vi "PS get status.vi"(8 "error in (no error)":errorcluster, 9 "Reset":bool, 11 "VISA Resource Name":refnum<visa-resource-name>) -> (0 "error out":errorcluster, 1 "Setpoint":dbl format="%.2f", 2 "Current":dbl(slide)=6.428571428571429 scale=-20.0..20.0 scale format="%.1f", 3 "dup VISA Resource Name":refnum<visa-resource-name>, 4 "Errors Out":string[](array[string]), 5 "Commands Out":string[](array[string]), 6 "% errors":dbl format="%.2f", 7 "Status":T1)   [LabVIEW 2020]
panel:
  out "Serial time":i32
  in  "samples lp filter":dbl
  out "execution time":dbl format="%.2f"
  out "# Errors":i32
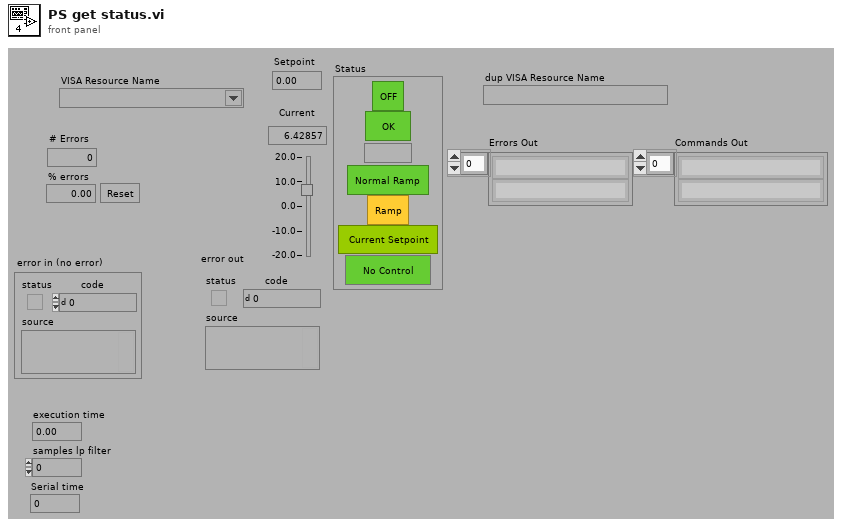
[diagram p1: front panel]
types:
  T1 = cluster{bool, bool, "Ramp Status":u16, bool, bool, bool, bool}
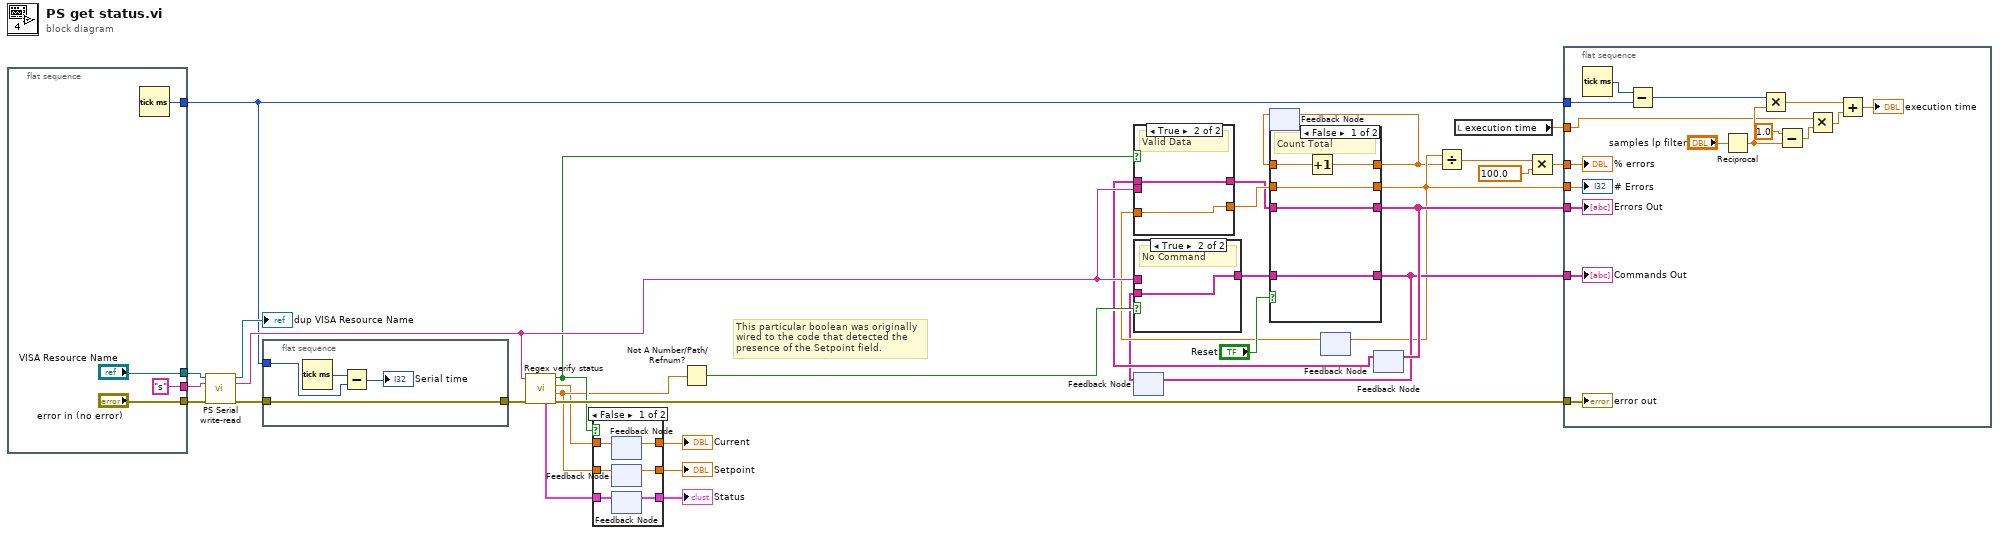
[diagram p0: block diagram]
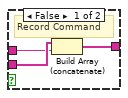
[diagram p2: hidden frame]
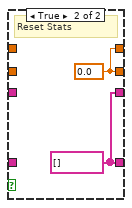
[diagram p3: hidden frame]
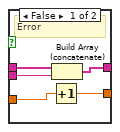
[diagram p4: hidden frame]
diagram:
  # "This particular boolean was originally\nwired to the code that detected the\npresence of the Setpoint field."
  n1 = flat-sequence {
    tunnel: ["s" ("String To Send")] -> w29
    tunnel: ["error in (no error)"] -> w28
    tunnel: ["VISA Resource Name"] -> w27
    tunnel: [w34] -> w20
    frame #0 {
      n2 = Tick Count (ms)() -> (millisecond timer value=w34:u32)
    }
  }
  n3 = call "PS Serial write-read.vi"("VISA Resource Name"=w27, "String To Send"=w29, "error in (no error)"=w28) -> ("dup VISA Resource Name"=→"dup VISA Resource Name":refnum<visa-resource-name>, "Serial Read"=w25:string, "error out"=w19:errorcluster)  [unwired: 8 in, 2 out]
  n4 = flat-sequence {
    tunnel: w20 -> [w39]
    tunnel: w19 -> [w38]
    tunnel: [w38] -> w18
    frame #0 {
      n5 = Tick Count (ms)() -> (millisecond timer value=w40:u32)
      n6 = Subtract(x=w40, y=w39) -> (x-y=→"Serial time":u32)
    }
  }
  n7 = call "Regex verify status.vi"("Error In"=w18, "Input String"=w25) -> ("Error Out"=w24:errorcluster, "Setpoint/Rate"=w4:dbl, "Current"=w2:dbl, "Valid Data"=w23:bool, "Status"=w6:T1)  [unwired: 5 in]
  n8 = case shown="False" w23 {
    tunnel: w2 -> [w47 w48]
    tunnel: w4 -> [w45 w49]
    tunnel: w6 -> [w44 w50]
    tunnel: [w42 w50] -> w5
    tunnel: [w43 w49] -> w3
    tunnel: [w46 w48] -> w1
    frame False {
      n9 = feedback-in #1(w47) -> ()
      n10 = feedback #1() -> (w46:dbl)  [unwired: 1 in]
      n11 = feedback-in #2(w45) -> ()
      n12 = feedback #2() -> (w43:dbl)  [unwired: 1 in]
      n13 = feedback-in #3(w44) -> ()
      n14 = feedback #3() -> (w42:T1)  [unwired: 1 in]
    }
    frame True {
    }
  }
  "Current" <- w1
  "Setpoint" <- w3
  "Status" <- w5
  n15 = Not A Number/Path/Refnum?(number/path/refnum=w4) -> (NaN/Path/Refnum?=w22:bool)
  n16 = feedback #4() -> (w8:string[])  [unwired: 1 in]
  n17 = case shown="True" w22 {
    tunnel: w8 -> [w53 w54]
    tunnel: [w52 w54] -> w7
    tunnel: w25 -> [w51 _]
    frame False {
      # "Record Command"
      n18 = Build Array (concatenate)(w53, w51) -> (w52:string[])
    }
    frame True {
      # "No Command"
    }
  }
  n19 = feedback #5() -> (w13:dbl)  [unwired: 1 in]
  n20 = feedback #6() -> (w12:dbl)  [unwired: 1 in]
  n21 = feedback #7() -> (w10:string[])  [unwired: 1 in]
  n22 = case shown="True" w23 {
    tunnel: [w58 w61] -> w11
    tunnel: w12 -> [w59 w61]
    tunnel: w10 -> [w56 w60]
    tunnel: [w57 w60] -> w9
    tunnel: w25 -> [w55 _]
    frame False {
      # "Error"
      n23 = Increment(x=w59) -> (x+1=w58:dbl)
      n24 = Build Array (concatenate)(w56, w55) -> (w57:string[])
    }
    frame True {
      # "Valid Data"
    }
  }
  n25 = case shown="False" "Reset" {
    tunnel: [w62 w68] -> w14
    tunnel: w13 -> [w66 _]
    tunnel: [w65 w68] -> w15
    tunnel: w11 -> [w65 _]
    tunnel: [w64 w67] -> w17
    tunnel: w9 -> [w64 _]
    tunnel: [w63 w67] -> w16
    tunnel: w7 -> [w63 _]
    frame False {
      # "Count Total"
      n26 = Increment(x=w66) -> (x+1=w62:dbl)
    }
    frame True {
      w67 = string[] []
      w68 = 0.0
      # "Reset Stats"
    }
  }
  n27 = feedback-in #4(w16) -> ()
  n28 = feedback-in #5(w14) -> ()
  n29 = feedback-in #6(w15) -> ()
  n30 = feedback-in #7(w17) -> ()
  n31 = Divide(x=w15, y=w14) -> (x/y=w33:dbl)
  n32 = local read "execution time"() -> (w21:dbl)
  n33 = Multiply(x=w33, y=100.0) -> (x*y=w31:dbl)
  n34 = flat-sequence {
    tunnel: w31 -> [w84]
    tunnel: w15 -> [w83]
    tunnel: w17 -> [w82]
    tunnel: w16 -> [w81]
    tunnel: w24 -> [w80]
    tunnel: w20 -> [w78]
    tunnel: w21 -> [w72]
    frame #0 {
      n35 = Tick Count (ms)() -> (millisecond timer value=w79:u32)
      n36 = Subtract(x=w79, y=w78) -> (x-y=w74:u32)
      n37 = Reciprocal(x="samples lp filter") -> (1/x=w75:dbl)
      n38 = Multiply(x=w74, y=w75) -> (x*y=w71:dbl)
      n39 = Subtract(x=1.0, y=w75) -> (x-y=w73:dbl)
      n40 = Multiply(x=w72, y=w73) -> (x*y=w70:dbl)
      n41 = Add(x=w71, y=w70) -> (x+y=→"execution time":dbl)
      "error out" <- w80
      "% errors" <- w84
      "# Errors" <- w83
      "Errors Out" <- w82
      "Commands Out" <- w81
    }
  }
